vi "COM.vi"(8 "error in (no error)":errorcluster, 10 "Command":string, 11 "VISA Refnum in":refnum<visa-resource-name>="COM3") -> (0 "error out":errorcluster, 2 "Response":string="\r\n", 3 "VISA Refnum out":refnum<visa-resource-name>)   [LabVIEW 2019, in "KH7008.lvlib"]
uses:
  KH7008.lvlib
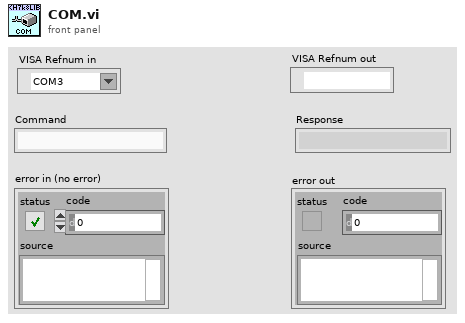
[diagram p1: front panel]
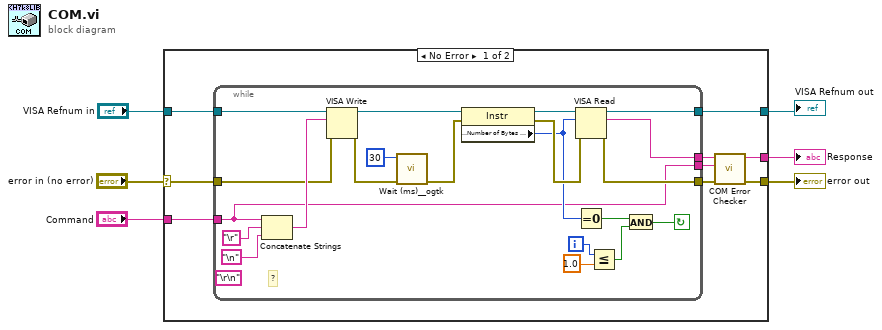
[diagram p0: block diagram]
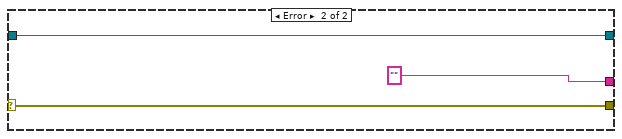
[diagram p2: hidden frame]
diagram:
  n1 = case shown="No Error" "error in (no error)" {
    selector: "error in (no error)" -> [w14 w37]
    tunnel: "VISA Refnum in" -> [w7 w38]
    tunnel: "Command" -> [w15 _]
    tunnel: [w12 w37] -> w3
    tunnel: [w11 "" ("String")] -> w2
    tunnel: [w9 w38] -> w1
    frame No Error {
      n2 = while {
        tunnel: w7 -> [w17]
        tunnel: w15 -> [w19]
        tunnel: w14 -> [w26]
        tunnel: [w32] -> w13
        tunnel: [w25] -> w10
        tunnel: [w18] -> w9
        tunnel: [w19] -> w8
        i -> [w30]
        stop <- w27 continue-if-true
        (unwired) "\r\n"
        # "?"
        n3 = Concatenate Strings(w19, "\r", "\n") -> (w36:string)
        n4 = VISA Write(VISA resource name=w17, write buffer=w36, error in (no error)=w26) -> (VISA resource name out=w34:refnum<visa-resource-name>, error out=w33:errorcluster)  [unwired: 1 out]
        n5 = call <userlib>:"Wait (ms)__ogtk.vi"("error in (no error)"=w33, "milliseconds to wait"=u32 30) -> ("error out"=w23:errorcluster)  [unwired: 8 in, 1 out]
        n6 = property class="Instr"(reference=w34, error in=w23) -> (reference out=w35:refnum<visa-resource-name>, error out=w21:errorcluster, "Serial Settings:Number of Bytes at Serial Port"=w20:u32)
        n7 = VISA Read(VISA resource name=w35, byte count=w20, error in (no error)=w21) -> (VISA resource name out=w18:refnum<visa-resource-name>, read buffer=w25:string, error out=w32:errorcluster)  [unwired: 1 out]
        n8 = Equal To 0?(x=w20) -> (x = 0?=w29:bool)
        n9 = Less Or Equal?(x=w30, y=1.0) -> (x <= y?=w28:bool)
        n10 = And(x=w29, y=w28) -> (x .and. y?=w27:bool)
      }
      n11 = call "COM Error Checker.vi"("error in (no error)"=w13, "Command"=w8, "Response"=w10) -> ("error out"=w12:errorcluster, "String"=w11:string)  [unwired: 7 in]
    }
    frame Error {
    }
  }
  "error out" <- w3
  "Response" <- w2
  "VISA Refnum out" <- w1
